vi "Execute.vi"(8 "error in (no error)":errorcluster, 11 "MyApp in":refnum<class "MyApp.lvclass">) -> (0 "error out":errorcluster, 3 "MyApp out":refnum<class "MyApp.lvclass">)   [LabVIEW 2012, in "MyApp.lvlib" / "MyApp.lvclass"]
uses:
  MyApp.lvclass
  HGF_LVC/HGF_BaseClasses/HGF_Event/HGF_Event.lvclass
  HGF_LVC/HGF_BaseClasses/HGF_Stop/HGF_Stop.lvclass
  <vilib>/Utility/error.llb/DialogType.ctl
  HGF_LVC/HGF_ApplicationBaseClasses/HGF_Application/HGF_Application.lvclass
panel:
  out "Iteration":i32
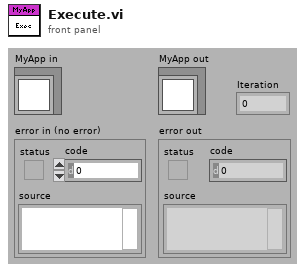
[diagram p1: front panel]
types:
  T1 = cluster{"seconds since 1Jan1904":timestamp, "message":string}
  T2 = typedef "DialogType.ctl" = u16
  T3 = cluster{"seconds since 1Jan1904":timestamp, string}
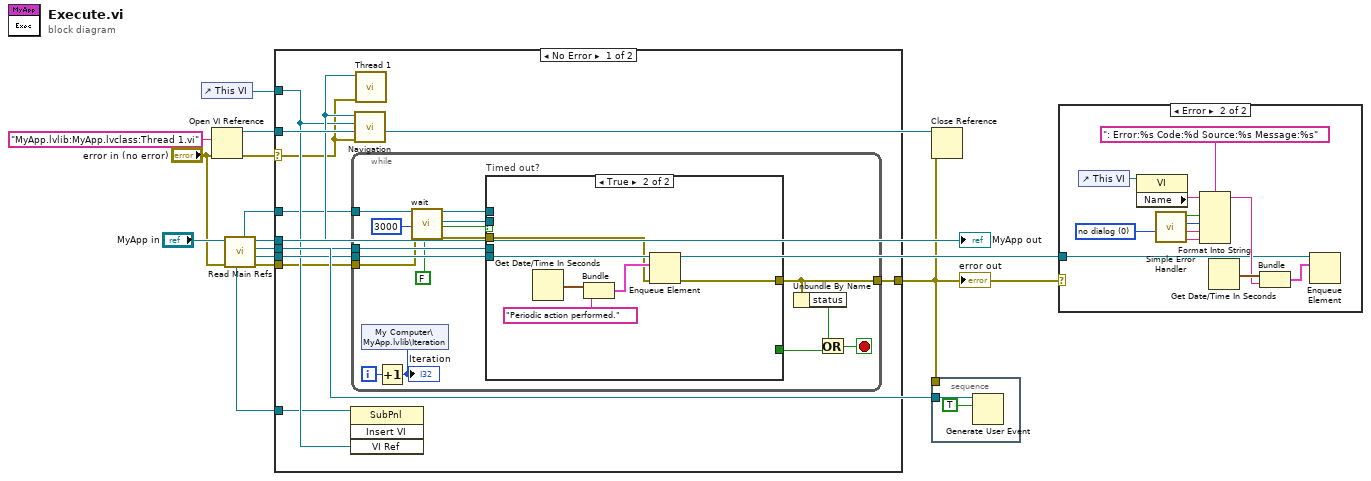
[diagram p0: block diagram]
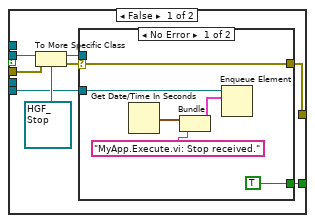
[diagram p3: hidden frame]
diagram:
  n1 = control-ref of="This VI"() -> (w9:refnum<vi>)
  n2 = Open VI Reference(vi path="MyApp.lvlib:MyApp.lvclass:Thread 1.vi", error in (no error)="error in (no error)") -> (vi reference=w8:refnum<vi>, error out=w4:errorcluster)  [unwired: 4 in]
  n3 = call "Read Main Refs.vi"("error in (no error)"="error in (no error)", "HGF_Application in"="MyApp in") -> ("error out"=w3:errorcluster, "Status Info Queue"=w2:refnum<queue>, "Main Stop Event"=w12:refnum<user-event>, "HGF_Application out"=w11:refnum<class "MyApp.lvclass">, "Info Event"=w7:refnum<class "HGF_Event.lvclass">, "Application Sub Panel"=w6:refnum<vi>)  [unwired: 2 in, 2 out]
  "MyApp out" <- w11
  n4 = case shown="No Error" w4 {
    selector: w4 -> [w15 w61]
    tunnel: w12 -> [w23 _]
    tunnel: w11 -> [w22 _]
    tunnel: w9 -> [w21 _]
    tunnel: w8 -> [w20 _]
    tunnel: [w19 w61] -> w1
    tunnel: w7 -> [w18 _]
    tunnel: w2 -> [w17 _]
    tunnel: w6 -> [w16 _]
    tunnel: w3 -> [w14 _]
    frame No Error {
      n5 = invoke class="SubPnl" method="Insert VI"(reference=w16, "VI Ref"=w21) -> ()  [unwired: 2 in, 4 out]
      n6 = while {
        tunnel: [w26] -> w19
        tunnel: w23 -> [w39]
        tunnel: w18 -> [w38]
        tunnel: w14 -> [w37]
        tunnel: w17 -> [w33]
        i -> [w29]
        stop <- w25 stop-if-true
        n7 = Increment(x=w29) -> (x+1=w28:i32)
        "Iteration" <- w28
        n8 = shared-variable "My Computer\\MyApp.lvlib\\Iteration"(w28) -> ()  [unwired: 1 in, 1 out]
        n9 = call-dynamic "wait.vi"("HGF_Event"=w38, "msTimeout (-1)"=3000, "error in (no error)"=w37, "ignore previous (F)"=FALSE) -> ("dup HGF_Event"=w34:refnum<class "HGF_Event.lvclass">, "Object"=w32:refnum<class>, "timed out"=w30:bool, "error out"=w35:errorcluster)  [unwired: 12 in]
        n10 = case "Timed out?" shown="True" w30 {
          tunnel: [w42 w55] -> w26
          tunnel: w39 -> [_ _]
          tunnel: w35 -> [w46 w56]
          tunnel: w34 -> [_ _]
          tunnel: w33 -> [w40 w58]
          tunnel: w32 -> [w47 _]
          tunnel: [w43 _] -> w31
          frame False {
            n11 = To More Specific Class(target class=refnum<class "HGF_Stop.lvclass"> refnum ("HGF_BaseClasses.lvlib:HGF_Stop.lvclass"), reference=w47, error in=w46) -> (specific class reference=w44:refnum<class "HGF_Stop.lvclass">, error out=w45:errorcluster)
            n12 = case shown="No Error" w45 {
              selector: w45 -> [w52 w54]
              tunnel: w44 -> [_ _]
              tunnel: [TRUE _] -> w43
              tunnel: [w52 w54] -> w42
              tunnel: w40 -> [w48 _]
              frame No Error {
                n13 = Get Date/Time In Seconds() -> (seconds since 1Jan1904=w50:timestamp)
                n14 = Bundle("seconds since 1Jan1904"=w50, "message"="MyApp.Execute.vi: Stop received.") -> (w51:T1)  [unwired: 1 in]
                n15 = Enqueue Element(queue=w48, element=w51) -> ()  [unwired: 2 in, 3 out]
              }
              frame Error {
              }
            }
          }
          frame True {
            n16 = Get Date/Time In Seconds() -> (seconds since 1Jan1904=w60:timestamp)
            n17 = Bundle("seconds since 1Jan1904"=w60, "message"="Periodic action performed.") -> (w57:T1)  [unwired: 1 in]
            n18 = Enqueue Element(queue=w58, element=w57, error in (no error)=w56) -> (error out=w55:errorcluster)  [unwired: 1 in, 2 out]
          }
        }
        n19 = Unbundle By Name(w26) -> ("status"=w24:bool)
        n20 = Or(x=w24, y=w31) -> (x .or. y?=w25:bool)
      }
      n21 = call "Navigation.vi"("error in (no error)"=w15, "Thread 1 Ref"=w20, "Thread 0 Ref"=w21, "MyApp in"=w22) -> ()  [unwired: 6 in, 2 out]
      n22 = call "Thread 1.vi"("error in (no error)"=w15, "MyApp in"=w22) -> ()  [unwired: 8 in, 2 out]
    }
    frame Error {
    }
  }
  "error out" <- w1
  n23 = Close Reference(reference=w8, error in (no error)=w1) -> ()  [unwired: 1 out]
  n24 = stacked-sequence {
    tunnel: w12 -> [w63]
    tunnel: w1 -> [_]
    frame #0 {
      n25 = Generate User Event(user event=w63, event data cluster=TRUE ("event data")) -> ()  [unwired: 1 in, 2 out]
    }
  }
  n26 = case shown="Error" w1 {
    tunnel: w2 -> [_ w64]
    frame No Error {
    }
    frame Error {
      w66 = T2 0 items=["no dialog", "OK message", "continue or stop message", "OK message + warnings", "continue/stop + warnings"] ("type of dialog (OK msg:1)")
      n27 = control-ref of="This VI"() -> (w65:refnum<vi>)
      n28 = property class="VI"(reference=w65) -> ("Name"=w73:string)  [unwired: 1 in, 2 out]
      n29 = call <vilib>:"Simple Error Handler.vi"("type of dialog (OK msg:1)"=w66) -> ("error?"=w72:bool, "code out"=w71:i32, "source out"=w70:string, "message"=w69:string)  [unwired: 4 in, 1 out]
      n30 = Format Into String(format string=": Error:%s Code:%d Source:%s Message:%s", initial string=w73, w72, w71, w70, w69) -> (resulting string=w67:string)  [unwired: 1 in, 1 out]
      n31 = Get Date/Time In Seconds() -> (seconds since 1Jan1904=w75:timestamp)
      n32 = Bundle("seconds since 1Jan1904"=w75, w67) -> (w74:T3)  [unwired: 1 in]
      n33 = Enqueue Element(queue=w64, element=w74) -> ()  [unwired: 2 in, 3 out]
    }
  }
